vi "Get VI Reference.vi"(8 "error in (no error)":errorcluster, 11 "SMO.UI_Embed In":refnum<class "SMO.UI_Embed.lvclass">) -> (0 "error out":errorcluster, 2 "VI Reference":refnum<vi>, 3 "SMO.UI_Embed Out":refnum<class "SMO.UI_Embed.lvclass">)   [LabVIEW 2013, in "SMO.UI_Embed.lvclass"]
uses:
  SMO.UI_Embed.lvclass
  <vilib>/JKI/JKI SMO/SMO/SMO.lvclass
panel:
  # "For instructions on how to use the JKI State Machine Objects, examples and video tutorials, visit:\nhttp://jki.net/state-machine-objects/\n\nJKI State Machine Objects™\nhttp://jki.net/state-machine-objects/\nCopyright (C) 2005-2015, JKI <info@jki.net>\nALL RIGHTS RESERVED"
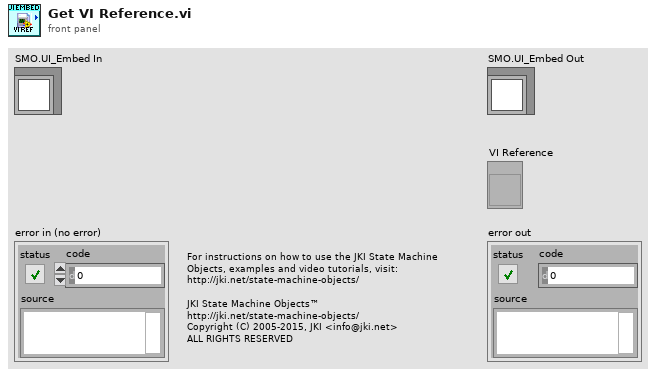
[diagram p1: front panel]
types:
  T1 = typedef "SMO.lvclass/RegisteredProcessData--Cluster.ctl" = cluster{"Name":string, "Static VI Ref":refnum<vi>, "Running":bool, "NotifierRef":u32}
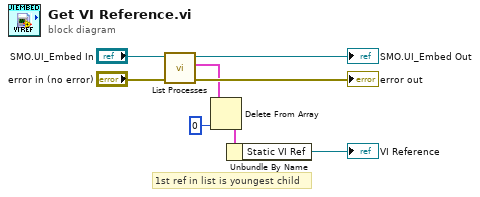
[diagram p0: block diagram]
diagram:
  # "1st ref in list is youngest child"
  n1 = call <vilib>:"List Processes.vi"("error in (no error)"="error in (no error)", "SMO"="SMO.UI_Embed In") -> ("error out"=→"error out":errorcluster, "Registered Processes"=w4:T1[], "SMO out"=→"SMO.UI_Embed Out":refnum<class "SMO.UI_Embed.lvclass">)  [unwired: 7 in]
  n2 = Delete From Array(array=w4, index=0) -> (deleted portion=w5:T1)  [unwired: 1 in, 1 out]
  n3 = Unbundle By Name(w5) -> ("Static VI Ref"=→"VI Reference":refnum<vi>)
